vi "move X Relative.vi"(10 "Speed X":i32, 11 "x mm":dbl) -> ()   [LabVIEW 2017]
uses:
  Settings/Traverse-Settings-Global.vi
  ICNC/ICNC2.lvlib
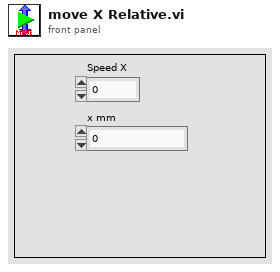
[diagram p1: front panel]
types:
  T1 = typedef "Settings-Control.ctl" = cluster{"Acceleration":dbl[], "Deceleration":dbl[], "Max Velocity":dbl[], "Speed":dbl, "Pulse/Degree":dbl, "Degre Factor":dbl[], "mm/rotation":dbl[], "Position":dbl[]}
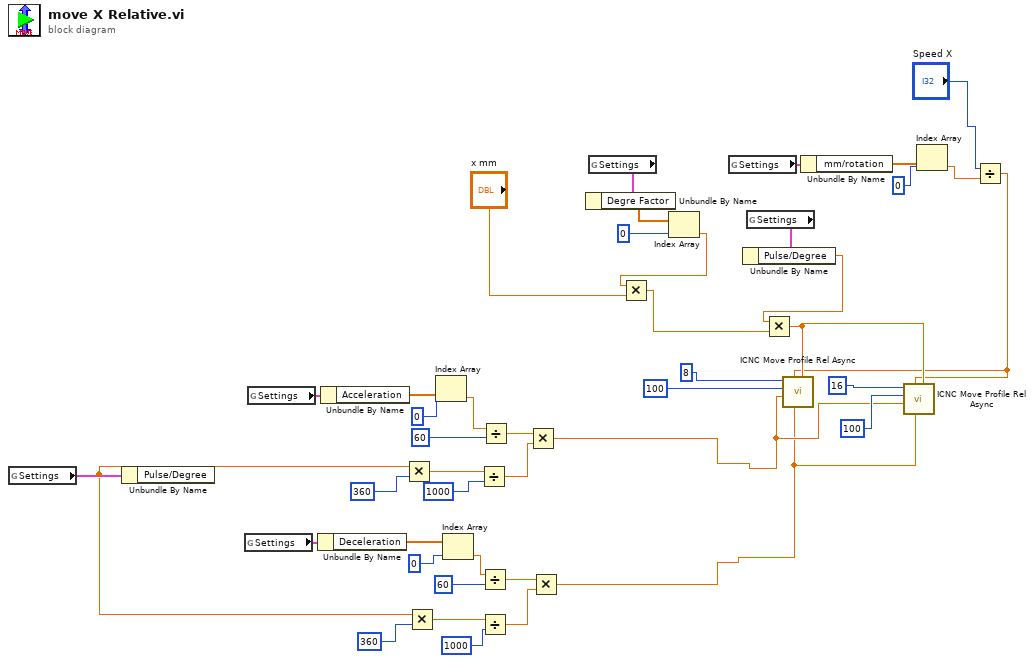
[diagram p0: block diagram]
diagram:
  n1 = global read "Traverse-Settings-Global.vi" "Settings"() -> (w25:T1)
  n2 = Unbundle By Name(w25) -> ("Pulse/Degree"=w24:dbl)
  n3 = global read "Traverse-Settings-Global.vi" "Settings"() -> (w20:T1)
  n4 = global read "Traverse-Settings-Global.vi" "Settings"() -> (w23:T1)
  n5 = Unbundle By Name(w20) -> ("Deceleration"=w19:dbl[])
  n6 = Unbundle By Name(w23) -> ("Acceleration"=w22:dbl[])
  n7 = Multiply(x=w24, y=360) -> (x*y=w33:dbl)
  n8 = Multiply(x=w24, y=360) -> (x*y=w32:dbl)
  n9 = Index Array(array=w22, index=0) -> (element=w11:dbl)
  n10 = Index Array(array=w19, index=0) -> (element=w10:dbl)
  n11 = Divide(x=w33, y=1000) -> (x/y=w43:dbl)
  n12 = Divide(x=w10, y=60) -> (x/y=w39:dbl)
  n13 = Divide(x=w32, y=1000) -> (x/y=w38:dbl)
  n14 = Divide(x=w11, y=60) -> (x/y=w34:dbl)
  n15 = Multiply(x=w34, y=w43) -> (x*y=w8:dbl)
  n16 = Multiply(x=w39, y=w38) -> (x*y=w7:dbl)
  n17 = global read "Traverse-Settings-Global.vi" "Settings"() -> (w15:T1)
  n18 = Unbundle By Name(w15) -> ("Degre Factor"=w12:dbl[])
  n19 = Index Array(array=w12, index=0) -> (element=w13:dbl)
  n20 = Multiply(x=w13, y="x mm") -> (x*y=w27:dbl)
  n21 = global read "Traverse-Settings-Global.vi" "Settings"() -> (w6:T1)
  n22 = global read "Traverse-Settings-Global.vi" "Settings"() -> (w17:T1)
  n23 = Unbundle By Name(w17) -> ("Pulse/Degree"=w16:dbl)
  n24 = Multiply(x=w16, y=w27) -> (x*y=w26:dbl)
  n25 = Unbundle By Name(w6) -> ("mm/rotation"=w5:dbl[])
  n26 = Index Array(array=w5, index=0) -> (element=w2:dbl)
  n27 = Divide(x="Speed X", y=w2) -> (x/y=w1:dbl)
  n28 = call <menus>:"ICNC Move Profile Rel Async.vi"("Distance"=w26, "Decel"=w7, "Speed"=w1, "Accel"=w8, "FStartStop"=100, "Axe"=8) -> ()  [unwired: 4 in, 2 out]
  n29 = call <menus>:"ICNC Move Profile Rel Async.vi"("Distance"=w26, "Decel"=w7, "Speed"=w1, "Accel"=w8, "FStartStop"=100, "Axe"=16) -> ()  [unwired: 4 in, 2 out]
